vi "Capture Edge Image (SubVI).vi"(0 "Data In":u8, 1 "Data Valid?":bool) -> (14 "Capture End?":bool)   [LabVIEW 2015]
uses:
  <vilib>/rvi/Emulation/niFpgaEmulationIsFPGAContextNoSignature.vi
  <vilib>/rvi/Emulation/niFpgaSctlEmulationGetInTimedLoop.vi
  <vilib>/rvi/errors/niFpgaSetErrorForExecOnDevCompSimple.vi
  <vilib>/rvi/eio/common/nirviEmuReportErrorAndStop.vi
  <vilib>/rvi/DataTransferAndStorage/Container/Common/niFpgaContainerGetUniqueNameForEmu.vi
  <vilib>/rvi/FIFO/Fifo_Resource/nirvififoEmulationSetSize.vi
  <vilib>/rvi/FIFO/Fifo_Resource/nirviFifoEmulationQueueMgr.vi
  <instcachedir>/0/nirviFifoEmulationQueueMgr_E5CAEC123FF24DC58D834DCA3CDAA9B5.lvgen/nirviFifoEmulationQueueMgr_E5CAEC123FF24DC58D834DCA3CDAA9B5_004.vi
  <vilib>/rvi/FIFO/Fifo_Resource/nirvififoEmulationDetermineInputValidOut.vi
  <vilib>/rvi/FIFO/Fifo_Resource/nirvififoEmulationCreateLock.vi
  <vilib>/rvi/Emulation/niFpgaProcessEmulError.vi
  <vilib>/rvi/FIFO/Fifo_Resource/nirvififoEmulationObtainLock.vi
  <vilib>/rvi/FIFO/Fifo_Resource/nirvififoEmulationReleaseLock.vi
  <vilib>/rvi/occurrence/nirviWaitOnOccurrenceBase.vi
  <vilib>/rvi/errors/nirviReportUnexpectedCaseInternalError.vi
  <vilib>/rvi/errors/nirviReportUnexpectedCaseInternalError (U32).vi
  <vilib>/rvi/DataTransferAndStorage/Container/XNode/niFpgaContainer.xnode
  <vilib>/rvi/FIFO/Fifo_Resource/nirvififoEmulationWrite.vi
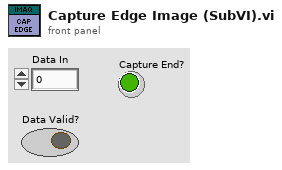
[diagram p1: front panel]
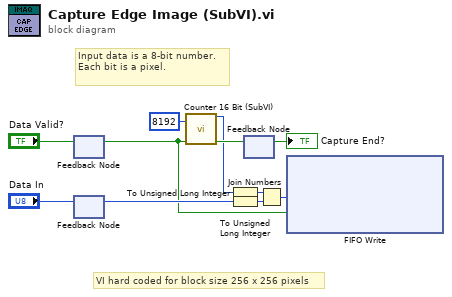
[diagram p0: block diagram]
diagram:
  # "VI hard coded for block size 256 x 256 pixels"
  # "Input data is a 8-bit number. Each bit is a pixel."
  n1 = feedback-in #1("Data Valid?") -> ()
  n2 = feedback #1() -> (w1:bool)  [unwired: 1 in]
  n3 = feedback-in #2("Data In") -> ()
  n4 = feedback #2() -> (w8:u8)  [unwired: 1 in]
  n5 = call "Counter 16 Bit (SubVI).vi"("Max. Count"=u16 8192, "Enable"=w1) -> ("Count"=w4:u16, "Count End?"=w9:bool)  [unwired: 11 in, 1 out]
  n6 = To Unsigned Long Integer(number=w4) -> (unsigned 32bit integer=w2:u32)
  n7 = To Unsigned Long Integer(number=w8) -> (unsigned 32bit integer=w6:u32)
  n8 = feedback-in #3(w9) -> ()
  n9 = feedback #3() -> (→"Capture End?":bool)  [unwired: 1 in]
  n10 = Join Numbers(hi=w2, lo=w6) -> ((hi.lo)=w5:u64)
  n11 = xnode ("FIFO Write")("Element"=w5, "Input Valid"=w1) -> ()  [unwired: 1 in, 2 out]
